vi "Get XPath.vi"   [LabVIEW 2016, in "SLL File IO.lvlib"]
doc: "For the given XPath expression, it returns the node text."
uses:
  SLL File IO.lvlib
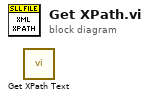
[diagram p0: block diagram]
diagram:
  n1 = call "Get XPath Text.vi"() -> ()  [unwired: 8 in, 4 out]
